vi "Pre Launch Init.vi"(11 "GUARDADOTEXTOPLANO in":refnum<class "GUARDADOTEXTOPLANO.lvclass">) -> (0 "error out":errorcluster, 3 "GUARDADOTEXTOPLANO out":refnum<class "GUARDADOTEXTOPLANO.lvclass">)   [LabVIEW 2019, in "GUARDADOTEXTOPLANO.lvlib" / "GUARDADOTEXTOPLANO.lvclass"]
doc: "(<B>Filename</B>: Actor Framework.lvlib:Actor.lvclass:Pre Launch Init.vi)\n\nDefines behavior that occurs after the Launch Nested Actor method is invoked but before the actor's Actor Core method begins running.\n\nBy default, this method does nothing. A descendant class may override it to define behavior."
uses:
  GUARDADOTEXTOPLANO.lvclass
  GUARDADOTEXTOPLANO.lvclass/GUARDADOTEXTOPLANO.ctl
  <vilib>/ActorFramework/Actor/Actor.lvclass
panel:
  in  "EXIT":bool=TRUE
  in  "GUARDAR?":bool=TRUE
  in  "DATO":string
  in  "PROVIENE DE?":enum16{"CONTADOR", "GENERADOR F"}(ring)
  in  "Path":path
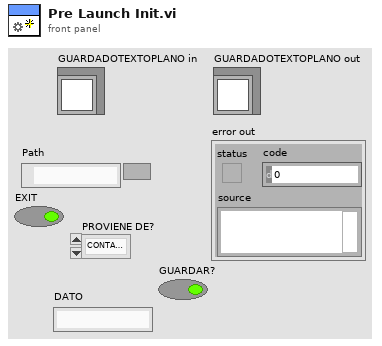
[diagram p1: front panel]
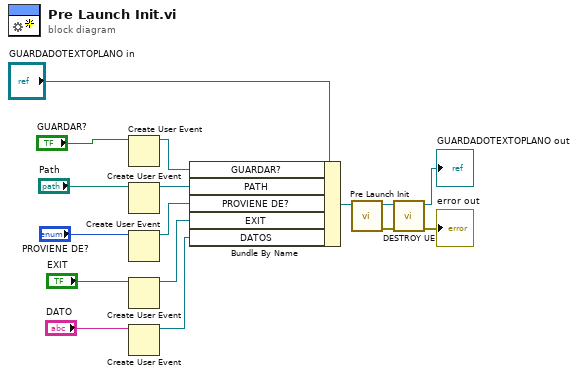
[diagram p0: block diagram]
diagram:
  n1 = Create User Event(user event datatype="GUARDAR?") -> (user event=w11:refnum<user-event>)  [unwired: 1 in, 1 out]
  n2 = Create User Event(user event datatype="Path") -> (user event=w10:refnum<user-event>)  [unwired: 1 in, 1 out]
  n3 = Create User Event(user event datatype="PROVIENE DE?") -> (user event=w9:refnum<user-event>)  [unwired: 1 in, 1 out]
  n4 = Create User Event(user event datatype="EXIT") -> (user event=w7:refnum<user-event>)  [unwired: 1 in, 1 out]
  n5 = Create User Event(user event datatype="DATO") -> (user event=w1:refnum<user-event>)  [unwired: 1 in, 1 out]
  n6 = Bundle By Name(cluster="GUARDADOTEXTOPLANO in", "GUARDAR?"=w11, "PATH"=w10, "PROVIENE DE?"=w9, "EXIT"=w7, "DATOS"=w1) -> (w12:refnum<class "GUARDADOTEXTOPLANO.lvclass">)
  n7 = call-parent "Pre Launch Init.vi"("Actor in"=w12) -> ("error out"=w6:errorcluster, "Actor out"=w5:refnum<class "GUARDADOTEXTOPLANO.lvclass">)  [unwired: 9 in]
  n8 = call "DESTROY UE.vi"("error in (no error)"=w6, "GUARDADOTEXTOPLANO in"=w5) -> ("error out"=→"error out":errorcluster, "GUARDADOTEXTOPLANO out"=→"GUARDADOTEXTOPLANO out":refnum<class "GUARDADOTEXTOPLANO.lvclass">)  [unwired: 8 in]
